vi "Impedance Correction.vi"() -> ()   [LabVIEW 2016]
uses:
  <vilib>/Utility/file.llb/Write Delimited Spreadsheet (DBL).vi
  <vilib>/Utility/file.llb/Read From Spreadsheet File (DBL).vi
panel:
  in  "Current Channels":string[](array[string])=["I X1 (Resampled)", "I Y1 (Resampled)"]
  in  "X channel":string="Field_fixed (Resampled)"
  in  "Group":string="p"
  in  "Signal Channels":string[](array[string])=["Vc1 X1 (Resampled)", "Vc1 Y1 (Resampled)"]
  in  "Save Button":bool
  in  "Chan #":i32=-1
  out "Current":cluster{"all rows":dbl[], dbl[]}[](graph)
  in  "Divide by current chan #":i32=-1
  in  "Fequency":dbl=300000.0 format="%#_6p"
  in  "stop":bool
  in  "V -> Impedance factor":dbl=100.0
  in  "C (parallel)":dbl(slide)=1e-09 step=1e-11 scale=0.0..5e-09 scale format="%#_6p"
  in  "L (series)":dbl(slide)=1e-15 scale=0.0..1e-12 scale format="%#_6p"
  in  "Phase":dbl(slide) step=0.1 scale=-180.0..180.0
  out "Data and Fix":cluster{"all rows":dbl[], dbl[]}[](graph)
  in  "Input file path":path
  # "=R_mon*GainI/GainV"
  # "Fix:  R=(I/V-Z_C^-1)^-1-Z_L"
  # "Column_X=chan # *2 +1\nColumn_Y=Column_X+1"
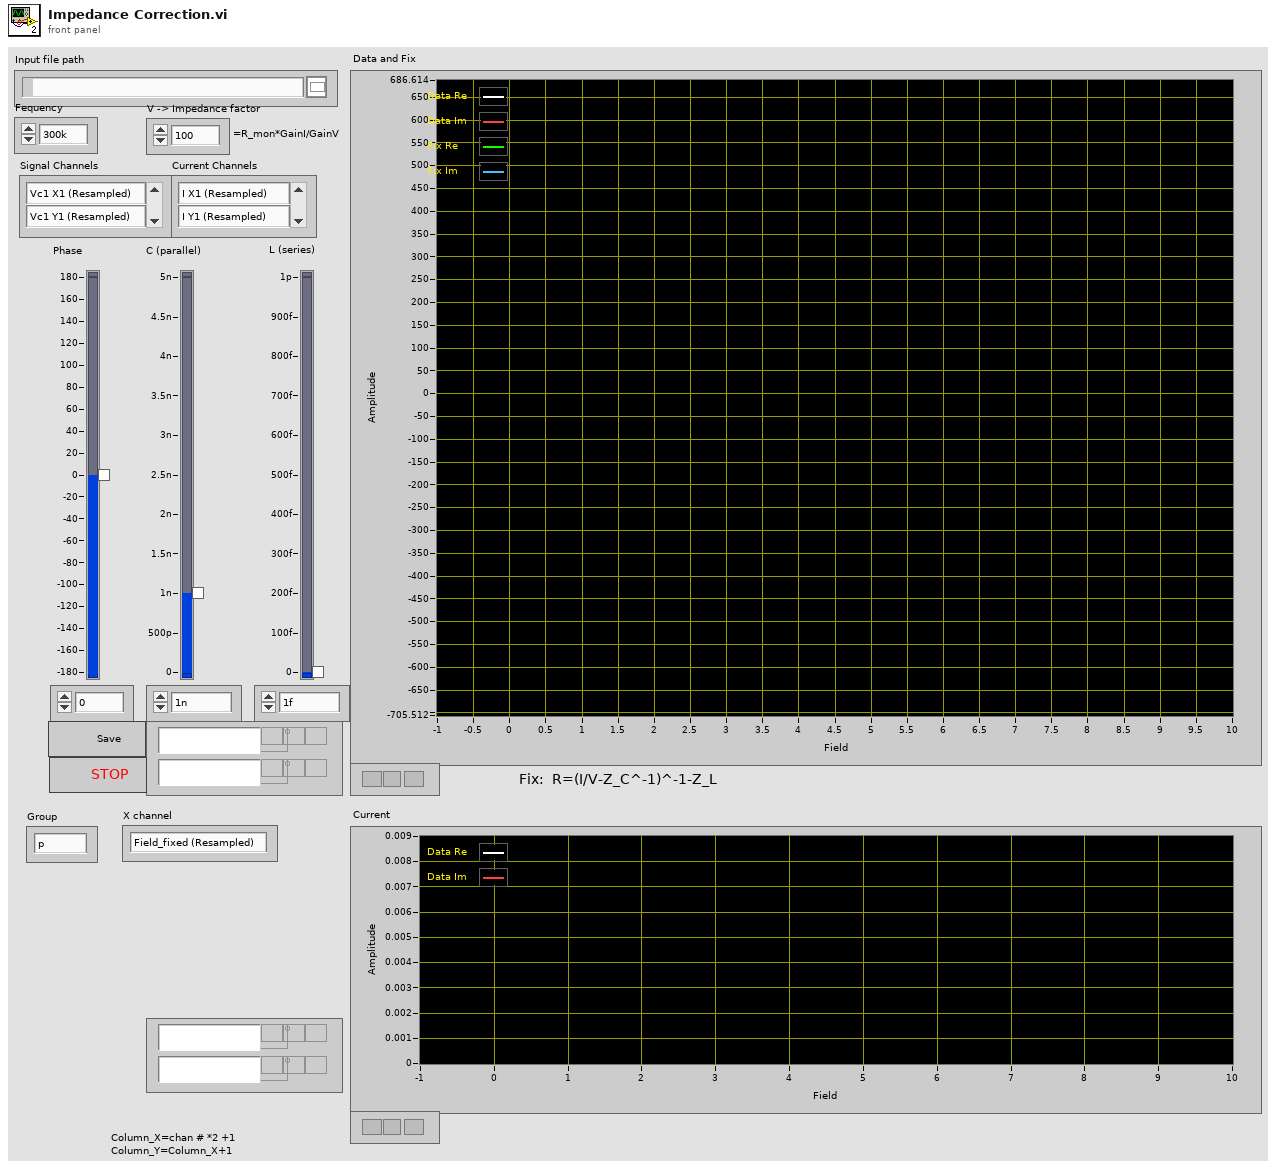
[diagram p1: front panel]
types:
  T1 = enum16{"open", "open or create", "create or replace", "create", "open (read-only)"}
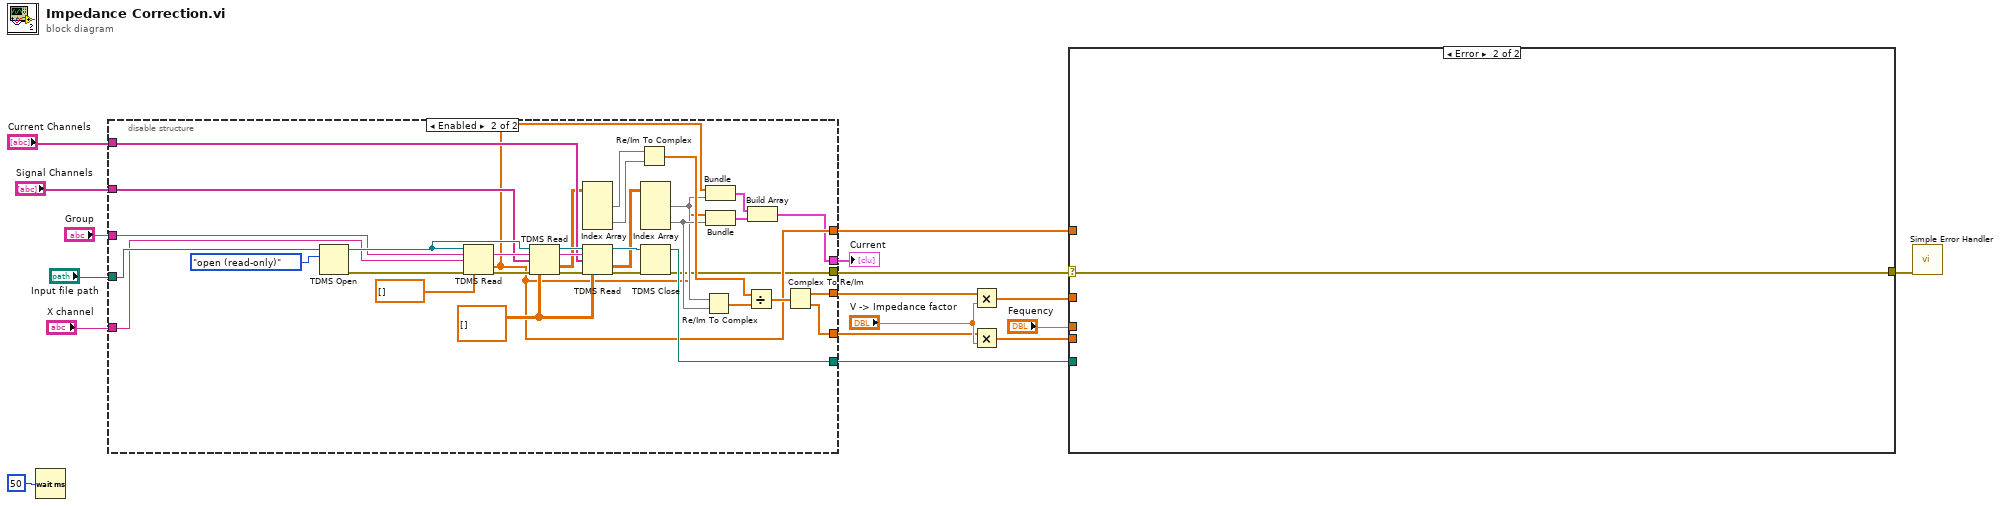
[diagram p0: block diagram]
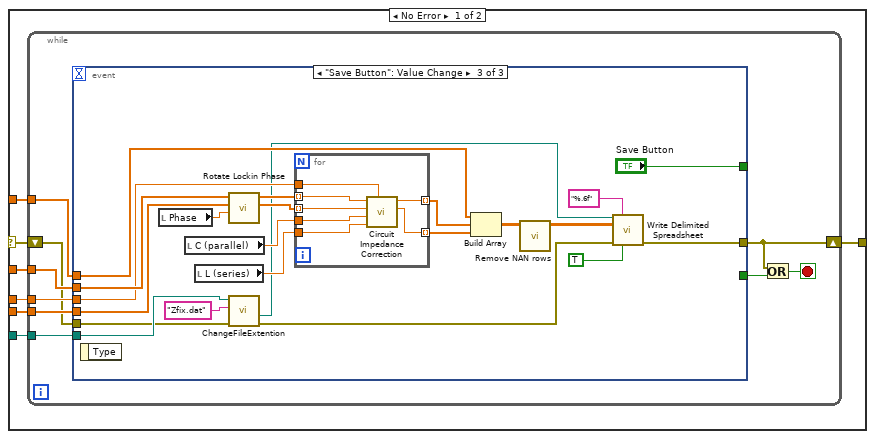
[diagram p2: hidden frame]
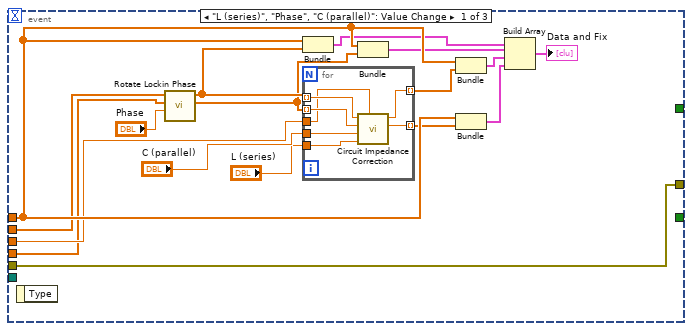
[diagram p3: hidden frame]
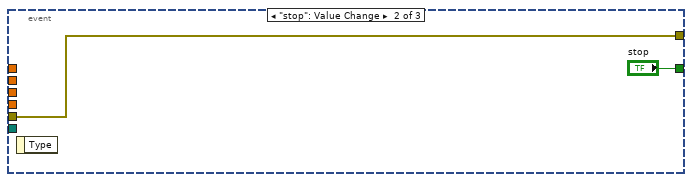
[diagram p4: hidden frame]
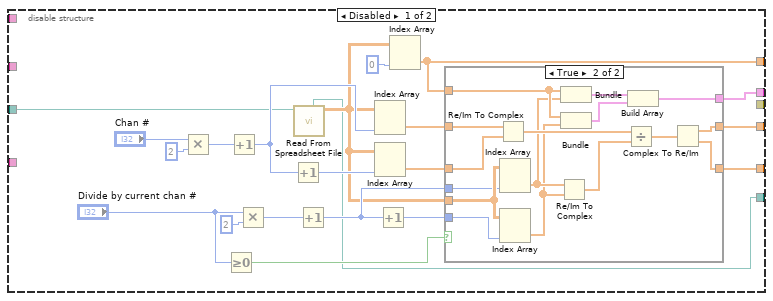
[diagram p5: hidden frame]
diagram:
  n1 = Wait (ms)(milliseconds to wait=u32 50) -> ()  [unwired: 1 out]
  n2 = disable-structure shown="Enabled" {
    disable-tunnel: [w36 w59] -> w13
    disable-tunnel: [w34 w58] -> w12
    disable-tunnel: [w27 w61] -> w11
    disable-tunnel: "Input file path" -> [w21 w81]
    disable-tunnel: [w19 w74] -> w8
    disable-tunnel: "Group" -> [_ w80]
    disable-tunnel: "X channel" -> [_ w79]
    disable-tunnel: "Signal Channels" -> [_ w78]
    disable-tunnel: "Current Channels" -> [_ w77]
    disable-tunnel: [w18 w60] -> w3
    disable-tunnel: [_ w57] -> w1
    frame Disabled {
      n3 = Multiply(x="Chan #", y=2) -> (x*y=w26:i32)
      n4 = Greater Or Equal To 0?(x="Divide by current chan #") -> (x >= 0?=w28:bool)
      n5 = Increment(x=w26) -> (x+1=w24:i32)
      n6 = Multiply(x="Divide by current chan #", y=2) -> (x*y=w31:i32)
      n7 = Increment(x=w24) -> (x+1=w23:i32)
      n8 = call-poly <vilib>:"Read From Spreadsheet File.vi"("file path (dialog if empty)"=w21) -> ("all rows"=w20:dbl[][], "new file path (Not A Path if cancelled)"=w19:path)  [unwired: 6 in, 3 out]
      n9 = Increment(x=w31) -> (x+1=w30:i32)
      n10 = Index Array(array=w20, index (col)=w24) -> (element=w37:dbl[])  [unwired: 1 in]
      n11 = Index Array(array=w20, index (col)=w23) -> (element=w35:dbl[])  [unwired: 1 in]
      n12 = Increment(x=w30) -> (x+1=w29:i32)
      n13 = Index Array(array=w20, index (col)=0 ("disabled index (col)")) -> (element=w27:dbl[])  [unwired: 1 in]
      n14 = case shown="True" w28 {
        tunnel: w37 -> [w40 w53]
        tunnel: [w40 w48] -> w36
        tunnel: w35 -> [w39 w52]
        tunnel: [w39 w47] -> w34
        tunnel: w20 -> [_ w56]
        tunnel: w30 -> [_ w55]
        tunnel: w29 -> [_ w54]
        tunnel: w27 -> [_ w44]
        tunnel: [_ w41] -> w18
        frame False {
        }
        frame True {
          n15 = Re/Im To Complex(1:w52, 2:w53) -> (0:w51:cdb[])
          n16 = Index Array(array=w56, index (col)=w55) -> (element=w43:dbl[])  [unwired: 1 in]
          n17 = Index Array(array=w56, index (col)=w54) -> (element=w42:dbl[])  [unwired: 1 in]
          n18 = Re/Im To Complex(1:w42, 2:w43) -> (0:w50:cdb[])
          n19 = Bundle("all rows"=w44, "all rows"=w43) -> (w46:cluster{"all rows":dbl[], "all rows":dbl[]})  [unwired: 1 in]
          n20 = Bundle("all rows"=w44, "all rows"=w42) -> (w45:cluster{"all rows":dbl[], "all rows":dbl[]})  [unwired: 1 in]
          n21 = Divide(x=w51, y=w50) -> (x/y=w49:cdb[])
          n22 = Build Array(w46, w45) -> (w41:cluster{"all rows":dbl[], "all rows":dbl[]}[])
          n23 = Complex To Re/Im(x + iy=w49) -> (x=w48:dbl[], y=w47:dbl[])
        }
      }
    }
    frame Enabled {
      w65 = dbl[][] [] ("all rows")
      n24 = TDMS Open(10:T1."open (read-only)" ("operation (0:open)"), 11:w81) -> (0:w86:errorcluster, 3:w88:refnum<k34>)  [unwired: 5 in]
      n25 = TDMS Read(0:w88, 5:w80, 7:w79, 11:w86, 12:dbl[] [] ("all rows")) -> (6:w89:string, 10:w61:dbl[], 15:w87:errorcluster)  [unwired: 3 in, 3 out]
      n26 = TDMS Read(0:w88, 5:w89, 7:w78, 11:w87, 12:w65) -> (4:w83:refnum<k34>, 6:w85:string, 10:w68:dbl[][], 15:w84:errorcluster)  [unwired: 3 in, 2 out]
      n27 = Index Array(array=w68) -> (element #1=w67:dbl[], element #2=w66:dbl[])  [unwired: 4 in]
      n28 = TDMS Read(0:w83, 5:w85, 7:w77, 11:w84, 12:w65) -> (4:w75:refnum<k34>, 10:w64:dbl[][], 15:w76:errorcluster)  [unwired: 3 in, 3 out]
      n29 = Re/Im To Complex(1:w66, 2:w67) -> (0:w73:cdb[])
      n30 = Index Array(array=w64) -> (element #1=w62:dbl[], element #2=w63:dbl[])  [unwired: 4 in]
      n31 = TDMS Close(8:w76, 11:w75) -> (0:w57:errorcluster, 3:w74:path)
      n32 = Re/Im To Complex(1:w63, 2:w62) -> (0:w72:cdb[])
      n33 = Bundle("all rows"=w61, "all rows"=w62) -> (w70:cluster{"all rows":dbl[], "all rows":dbl[]})  [unwired: 1 in]
      n34 = Bundle("all rows"=w61, "all rows"=w63) -> (w69:cluster{"all rows":dbl[], "all rows":dbl[]})  [unwired: 1 in]
      n35 = Divide(x=w73, y=w72) -> (x/y=w71:cdb[])
      n36 = Build Array(w70, w69) -> (w60:cluster{"all rows":dbl[], "all rows":dbl[]}[])
      n37 = Complex To Re/Im(x + iy=w71) -> (x=w59:dbl[], y=w58:dbl[])
    }
  }
  "Current" <- w3
  n38 = Multiply(x=w13, y="V -> Impedance factor") -> (x*y=w17:dbl[])
  n39 = Multiply(x=w12, y="V -> Impedance factor") -> (x*y=w16:dbl[])
  n40 = case shown="Error" w1 {
    selector: w1 -> [w91 w162]
    tunnel: w17 -> [w97 _]
    tunnel: w16 -> [w96 _]
    tunnel: "Fequency" -> [w95 _]
    tunnel: w11 -> [w94 _]
    tunnel: w8 -> [w93 _]
    tunnel: [w92 w162] -> w2
    frame No Error {
      n41 = while {
        tunnel: w97 -> [w103]
        tunnel: w96 -> [w102]
        tunnel: w94 -> [w106]
        tunnel: w95 -> [w104]
        tunnel: w93 -> [w101]
        shift-right: [w98] -> w92
        shift-left: w91 -> [w100]
        stop <- w99 stop-if-true
        n42 = event shown="[2] \"Save Button\": Value Change" {
          selector: _ -> [_ _ _]
          dyn-events: _ -> [_ _ _]
          timeout: _ -> [_ _ _]
          tunnel: w106 -> [w123 _ w143]
          tunnel: [_ "stop" _] -> w105
          tunnel: w104 -> [w119 _ w146]
          tunnel: w103 -> [w111 _ w150]
          tunnel: w102 -> [w109 _ w149]
          tunnel: [_ _ "Save Button"] -> _
          tunnel: w101 -> [_ _ w144]
          tunnel: w100 -> [w107 w131 w135]
          tunnel: [w107 w131 w133] -> w98
          event "L (series)", "Phase", "C (parallel)": Value Change {
            n43 = event-data() -> ()  [unwired: 1 in, 1 out]
            n44 = call "Rotate Lockin Phase.vi"("Phase"="Phase", "Array Y in"=w109, "Array X in"=w111) -> ("Array Y out"=w108:dbl[], "Array X out"=w110:dbl[])  [unwired: 7 out]
            n45 = Bundle("all rows"=w123, "Array X out"=w110) -> (w122:cluster{"all rows":dbl[], "Array X out":dbl[]})  [unwired: 1 in]
            n46 = for {
              tunnel: w110 -> [w130] mode=indexing
              tunnel: w108 -> [w129] mode=indexing
              tunnel: "C (parallel)" -> [w128]
              tunnel: w119 -> [w127]
              tunnel: "L (series)" -> [w126]
              tunnel: [w125] -> w117 mode=indexing
              tunnel: [w124] -> w116 mode=indexing
              n47 = call "Circuit Impedance Correction.vi"("Fequency"=w127, "Series inductance"=w126, "Parallel capacitance"=w128, "Measured Resistance Y"=w129, "Measured Resistance X"=w130) -> ("Corrected resistance Y"=w124:dbl, "Corrected resistance X"=w125:dbl)  [unwired: 4 in, 1 out]
            }
            n48 = Bundle("all rows"=w123, "Array Y out"=w108) -> (w121:cluster{"all rows":dbl[], "Array Y out":dbl[]})  [unwired: 1 in]
            n49 = Bundle("all rows"=w123, w117) -> (w115:cluster{"all rows":dbl[], dbl[]})  [unwired: 1 in]
            n50 = Bundle("all rows"=w123, w116) -> (w114:cluster{"all rows":dbl[], dbl[]})  [unwired: 1 in]
            n51 = Build Array(w122, w121, w115, w114) -> (→"Data and Fix":cluster{"all rows":dbl[], "Array Y out":dbl[]}[])
          }
          event "stop": Value Change {
            n52 = event-data() -> ()  [unwired: 1 in, 1 out]
          }
          event "Save Button": Value Change {
            n53 = event-data() -> ()  [unwired: 1 in, 1 out]
            n54 = local read "Phase"() -> (w151:dbl)
            n55 = local read "C (parallel)"() -> (w147:dbl)
            n56 = local read "L (series)"() -> (w148:dbl)
            n57 = call "Rotate Lockin Phase.vi"("Phase"=w151, "Array Y in"=w149, "Array X in"=w150) -> ("Array Y out"=w152:dbl[], "Array X out"=w153:dbl[])  [unwired: 7 out]
            n58 = call "ChangeFileExtention.vi"("Error In"=w135, "New extension"="Zfix.dat" ("New Extention"), "File Path"=w144) -> ("Error Out"=w134:errorcluster, "Path with new extension"=w138:path)  [unwired: 1 in, 6 out]
            n59 = for {
              tunnel: w153 -> [w161] mode=indexing
              tunnel: w152 -> [w160] mode=indexing
              tunnel: w147 -> [w159]
              tunnel: w146 -> [w158]
              tunnel: w148 -> [w157]
              tunnel: [w156] -> w142 mode=indexing
              tunnel: [w155] -> w141 mode=indexing
              n60 = call "Circuit Impedance Correction.vi"("Fequency"=w158, "Series inductance"=w157, "Parallel capacitance"=w159, "Measured Resistance Y"=w160, "Measured Resistance X"=w161) -> ("Corrected resistance Y"=w155:dbl, "Corrected resistance X"=w156:dbl)  [unwired: 4 in, 1 out]
            }
            n61 = Build Array(w143, w142, w141) -> (w140:dbl[][])
            n62 = call "Remove NAN rows.vi"("Array - Numeric"=w140) -> ("Array out"=w137:dbl[][])  [unwired: 10 in]
            n63 = call-poly <vilib>:"Write Delimited Spreadsheet.vi"("file path (dialog if empty)"=w138, "format (%.3f)"="%.6f", "2D data"=w137, "error in (no error)"=w134, "transpose? (no:F)"=TRUE) -> ("error out"=w133:errorcluster)  [unwired: 9 in, 1 out]
          }
        }
        n64 = Or(x=w98, y=w105) -> (x .or. y?=w99:bool)
      }
    }
    frame Error {
    }
  }
  n65 = call <vilib>:"Simple Error Handler.vi"("error in (no error)"=w2) -> ()  [unwired: 4 in, 5 out]
